vi "DTbl Digital Size.vi"(8 "error in (no error)":errorcluster caption="错误输入（无错误）", 11 "digital data in":digitaldata caption="数字数据输入") -> (0 "error out":errorcluster caption="错误输出", 1 "number of signals":i32 caption="信号数", 2 "number of samples":i32 caption="采样数", 3 "digital data out":digitaldata caption="数字数据输出")   [LabVIEW 2018]
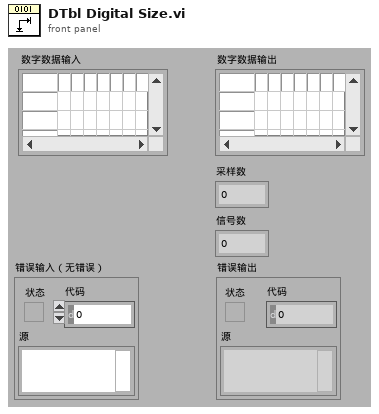
[diagram p1: front panel]
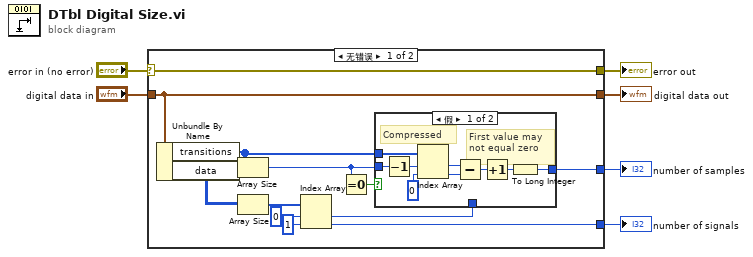
[diagram p0: block diagram]
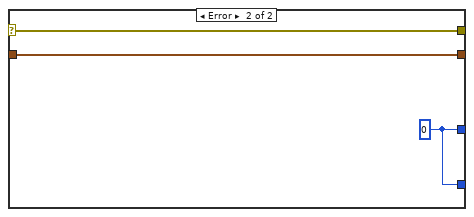
[diagram p3: hidden frame]
diagram:
  n1 = case shown="无错误" "error in (no error)" {
    selector: "error in (no error)" -> [w9 w31]
    tunnel: "digital data in" -> [w16 w29]
    tunnel: [w16 w29] -> w5
    tunnel: [w14 w30] -> w6
    tunnel: [w9 w31] -> w3
    tunnel: [w12 w30] -> w1
    frame No Error {
      n2 = Unbundle By Name(w16) -> ("transitions"=w10:u32[], "data"=w11:u8[][])
      n3 = Array Size(array=w10) -> (size(s)=w7:i32)
      n4 = Array Size(array=w11) -> (size(s)=w17:i32[])
      n5 = Index Array(array=w17, index #1=0 ("Index"), index #2=1 ("Index")) -> (element #1=w8:i32, element #2=w14:i32)
      n6 = Equal To 0?(x=w7) -> (x = 0?=w13:bool)
      n7 = case shown="假" w13 {
        tunnel: w10 -> [w27 _]
        tunnel: w7 -> [w26 _]
        tunnel: [w23 w28] -> w12
        tunnel: w8 -> [_ w28]
        frame False {
          # "Compressed"
          # "First value may\nnot equal zero"
          n8 = Decrement(x=w26) -> (x-1=w25:i32)
          n9 = Index Array(array=w27, index #1=w25, index #2=0 ("Index")) -> (element #1=w20:u32, element #2=w21:u32)
          n10 = Subtract(x=w20, y=w21) -> (x-y=w19:u32)
          n11 = Increment(x=w19) -> (x+1=w24:u32)
          n12 = To Long Integer(number=w24) -> (32bit integer=w23:i32)
        }
        frame True {
          # "Uncompressed"
        }
      }
    }
    frame Error {
      w30 = 0
    }
  }
  "number of signals" <- w6
  "digital data out" <- w5
  "error out" <- w3
  "number of samples" <- w1
